vi "WriteFiles.vi"(8 "error in (no error)":errorcluster, 11 "Master in":refnum<class "Master.lvclass">) -> (0 "error out":errorcluster, 3 "Master out":refnum<class "Master.lvclass">)   [LabVIEW 2014, in "Master.lvclass"]
uses:
  Master/Master.lvclass
  Master/Master.lvclass/Master.ctl
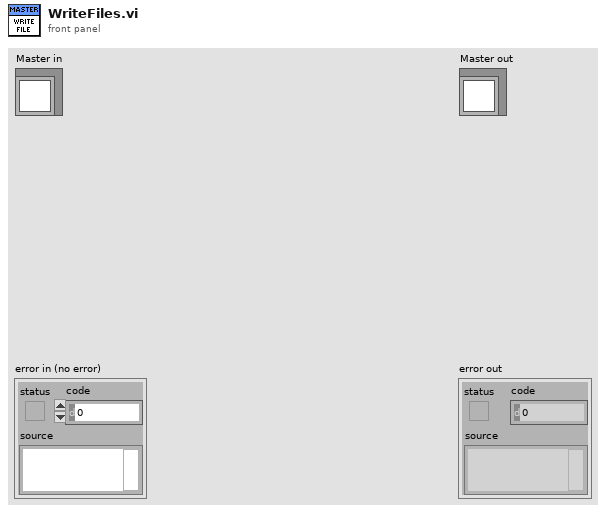
[diagram p1: front panel]
types:
  T1 = enum16{"open", "replace", "create", "open or create", "replace or create", "replace or create with confirmation"}
  T2 = cluster{"type string":i16[], "data string":string}
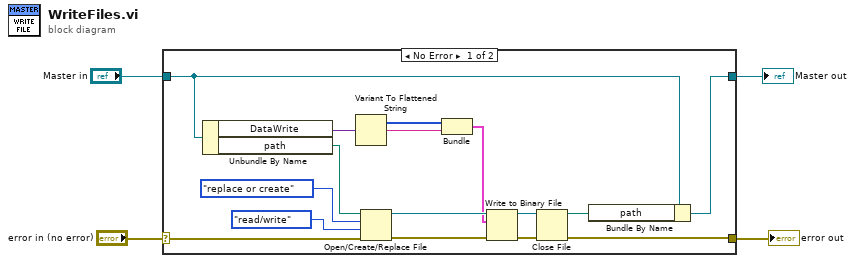
[diagram p0: block diagram]
diagram:
  n1 = case shown="No Error" "error in (no error)" {
    selector: "error in (no error)" -> [w17 w22]
    tunnel: [w12 w22] -> w3
    tunnel: [w7 w21] -> w1
    tunnel: "Master in" -> [w8 w21]
    frame No Error {
      n2 = Unbundle By Name(w8) -> ("DataWrite"=w9:variant, "path"=w20:path)
      n3 = Variant To Flattened String(Variant=w9) -> (data string=w11:string, 1:w5:i16[])
      n4 = Open/Create/Replace File(file path (use dialog)=w20, error in=w17, operation (0:open)=T1."replace or create", access (0:read/write)=enum16{"read/write", "read-only", "write-only"}."read/write") -> (refnum out=w16:refnum<file>, error out=w15:errorcluster)  [unwired: 2 in, 1 out]
      n5 = Bundle("type string"=w5, "data string"=w11) -> (w10:T2)  [unwired: 1 in]
      n6 = Write to Binary File(file (use dialog)=w16, data=w10, error in=w15) -> (refnum out=w14:refnum<file>, error out=w13:errorcluster)  [unwired: 3 in, 1 out]
      n7 = Close File(refnum=w14, error in=w13) -> (path=w6:path, error out=w12:errorcluster)
      n8 = Bundle By Name(cluster=w8, "path"=w6) -> (w7:refnum<class "Master.lvclass">)
    }
    frame Error {
    }
  }
  "error out" <- w3
  "Master out" <- w1
